vi "Read User Tag.vi"(8 "error in":errorcluster, 11 "Has Timestamp in":refnum<class "Has Time Stamp.lvclass">) -> (0 "error out":errorcluster, 2 "user tag":i32, 3 "Has Timestamp out":refnum<class "Has Time Stamp.lvclass">)   [LabVIEW 2020, in "PV Access.lvlib" / "PV Data.lvlib" / "Has Time Stamp.lvclass"]
uses:
  Has Time Stamp.lvclass
  3a2aeaae-d079-45d7-aa80-7f158ca5949c.vi
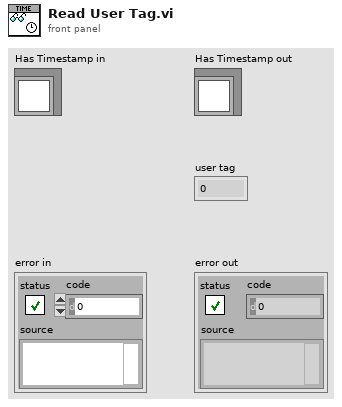
[diagram p1: front panel]
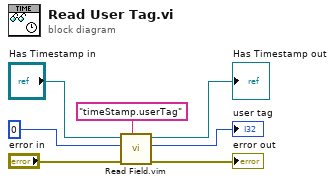
[diagram p0: block diagram]
diagram:
  n1 = call "Read Field.vim"("field"="timeStamp.userTag" ("element name"), "error in"="error in", "default value"=0, "Base Interface in"="Has Timestamp in") -> ("error out"=→"error out":errorcluster, "value"=→"user tag":i32, "Base Interface out"=→"Has Timestamp out":refnum<class "Has Time Stamp.lvclass">)  [unwired: 5 in]
